vi "Lidar Read.vi"(7 "error in (no error)":errorcluster, 10 "VISA resource name":refnum<visa-resource-name>) -> (0 "error out":errorcluster, 1 "Visual Out":cluster{dbl[], dbl[]}, 2 "XY Array":T2, 3 "VISA resource name out":refnum<visa-resource-name>)   [LabVIEW 2017]
uses:
  040-typeDefs/LidarPoint.ctl
  050-Tests/Wall Following/XY.ctl
  <instrlib>/Hokuyo URG Series/Hokuyo URG Series.lvlib
panel:
  in  "Array":T1[](array[typedef])
  in  "XY":T1
  out "XY Graph":cluster{"Y":dbl[], "Y":dbl[]}[](graph)
  in  "Encoding Width":u16(ring)=3 items=["2 Byte"=2, "3 Byte"=3]
  in  "Cluster Count":dbl=1.0
  in  "Start Point":dbl=-120.0
  in  "End Point":dbl=120.0
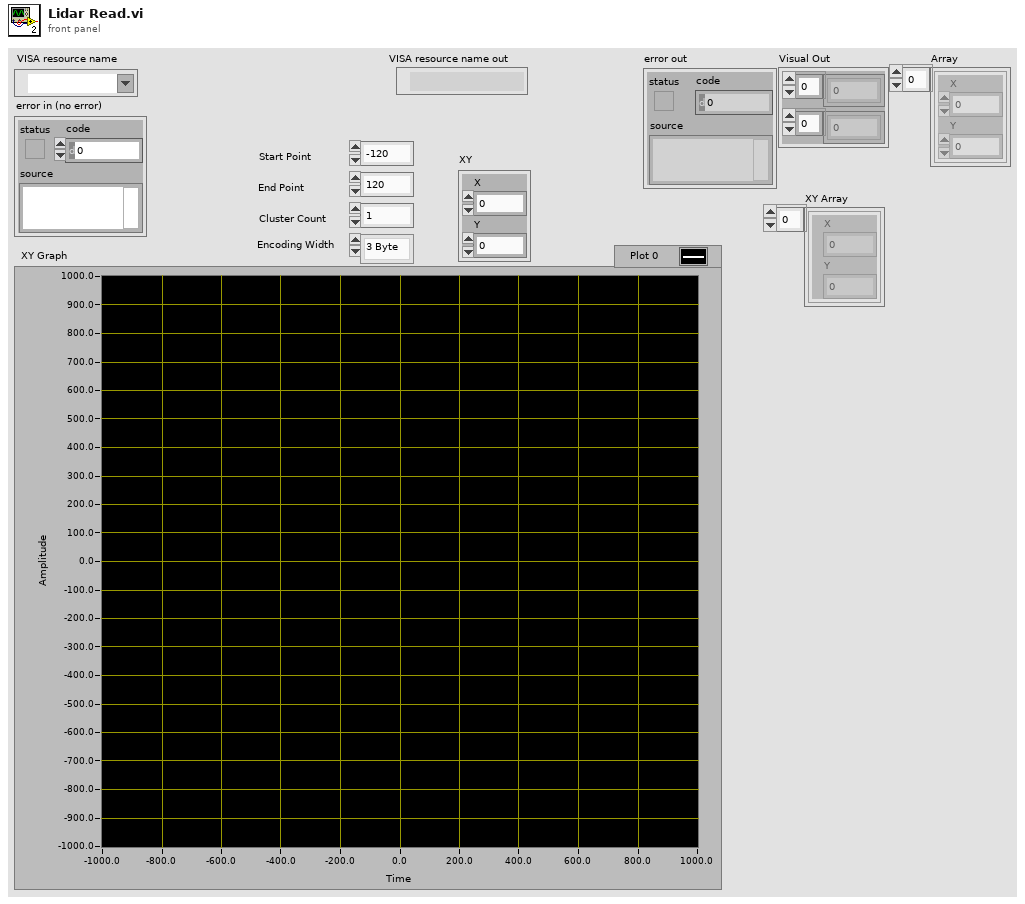
[diagram p1: front panel]
types:
  T1 = typedef "LidarPoint.ctl" = cluster{"X":dbl, "Y":dbl}
  T2 = typedef "XY.ctl" = T1[]
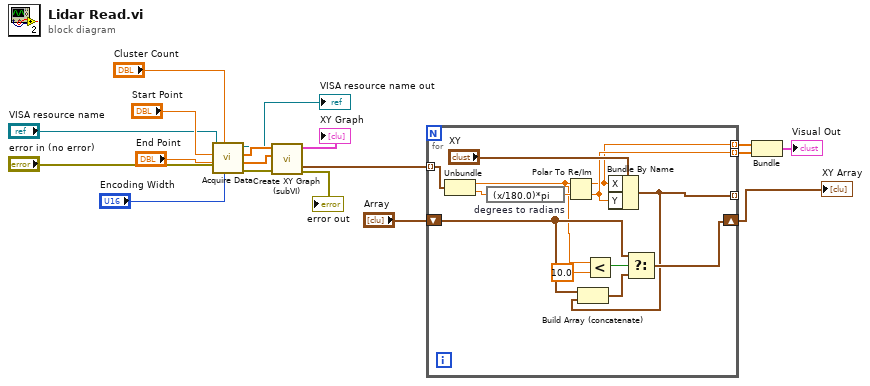
[diagram p0: block diagram]
diagram:
  n1 = call <instrlib>:"Acquire Data.vi"("Data Encoding Width (3 Byte)"="Encoding Width", "Cluster Count (1)"="Cluster Count", "error in (no error)"="error in (no error)", "End Point (120°)"="End Point", "Start Point (-120°)"="Start Point", "VISA resource name"="VISA resource name") -> ("error out"=w12:errorcluster, "Direction"=w13:dbl[], "Magnitude"=w14:dbl[], "VISA resource name out"=→"VISA resource name out":refnum<visa-resource-name>)  [unwired: 2 in]
  n2 = call "Create XY Graph (subVI).vi"("error in"=w12, "Direction"=w13, "Magnitude"=w14) -> ("error out"=→"error out":errorcluster, "Polar Array"=w6:cluster{dbl, dbl}[], "XY Graph"=→"XY Graph":cluster{"Y":dbl[], "Y":dbl[]}[])  [unwired: 6 in]
  n3 = for {
    tunnel: w6 -> [w31] mode=indexing
    tunnel: [w22] -> _ mode=indexing
    tunnel: [w26] -> w5 mode=indexing
    tunnel: [w27] -> w4 mode=indexing
    shift-right: [w25] -> w1
    shift-left: "Array" -> [w23]
    n4 = Unbundle(w31) -> (w21:dbl, w28:dbl)
    n5 = expression code="(x/180.0)*pi" "degrees to radians"(w28) -> (w29:dbl)
    n6 = Polar To Re/Im(2:w29, 3:w21) -> (0:w27:dbl, 1:w26:dbl)
    n7 = Less?(x=w21, y=10.0) -> (x < y?=w20:bool)
    n8 = Bundle By Name(cluster="XY", "X"=w26, "Y"=w27) -> (w22:T1)
    n9 = Build Array (concatenate)(w23, w22) -> (w24:T1[])
    n10 = Select(t=w23, s=w20, f=w24) -> (s? t:f=w25:T1[])
  }
  "XY Array" <- w1
  n11 = Bundle(w5, w4) -> (→"Visual Out":cluster{dbl[], dbl[]})  [unwired: 1 in]
